vi "Settings_dialog.vi"(11 "Initial_cofig":path) -> (1 "canceled or no change?":bool, 3 "Settings":T1)   [LabVIEW 2012]
uses:
  controls/Video_analizer_settings.ctl
  <vilib>/Utility/config.llb/Read Key (Double).vi
  <vilib>/Utility/config.llb/Read Key (Boolean).vi
  <vilib>/Utility/config.llb/Read Key (U32).vi
  <vilib>/Utility/config.llb/NI_LVConfig.lvlib
panel:
  in  "Order":u32 caption="Порядок"
  in  "Cutof_freq":dbl caption="Частота среза, Гц"
  in  "FIR_enable":bool caption="Вкл. цифровой фильтр"
  in  "VoltageY_offset":dbl caption="Смещение по Y напряжения, В"
  in  "CurrentY_offset":dbl caption="Смещение по Y тока, А"
  in  "Video_shift_in":dbl caption="Смещение видео-напряжение, мкс" min=0.0
  in  "Current_shift_in":dbl caption="Смещение ток-напряжение, мкс" min=0.0
  in  "Cancel Button":bool
  in  "Save Button":bool
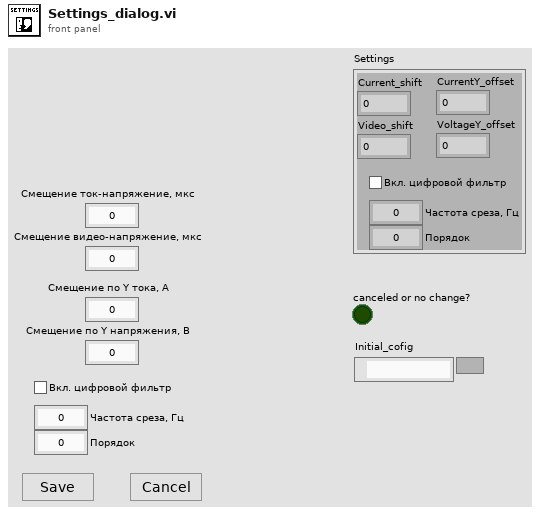
[diagram p1: front panel]
types:
  T1 = typedef "Video_analizer_settings.ctl" = cluster{"Current_shift":dbl, "Video_shift":dbl, "CurrentY_offset":dbl, "VoltageY_offset":dbl, "FIR_enable":bool, "Cutof_freq":dbl, "Order":u32}
  T2 = typedef "NI_LVConfig.lvlib/Config Data RefNum.ctl" = refnum<k1>
  T3 = enum8{"Enabled", "Disabled", "Disabled and Grayed Out"}
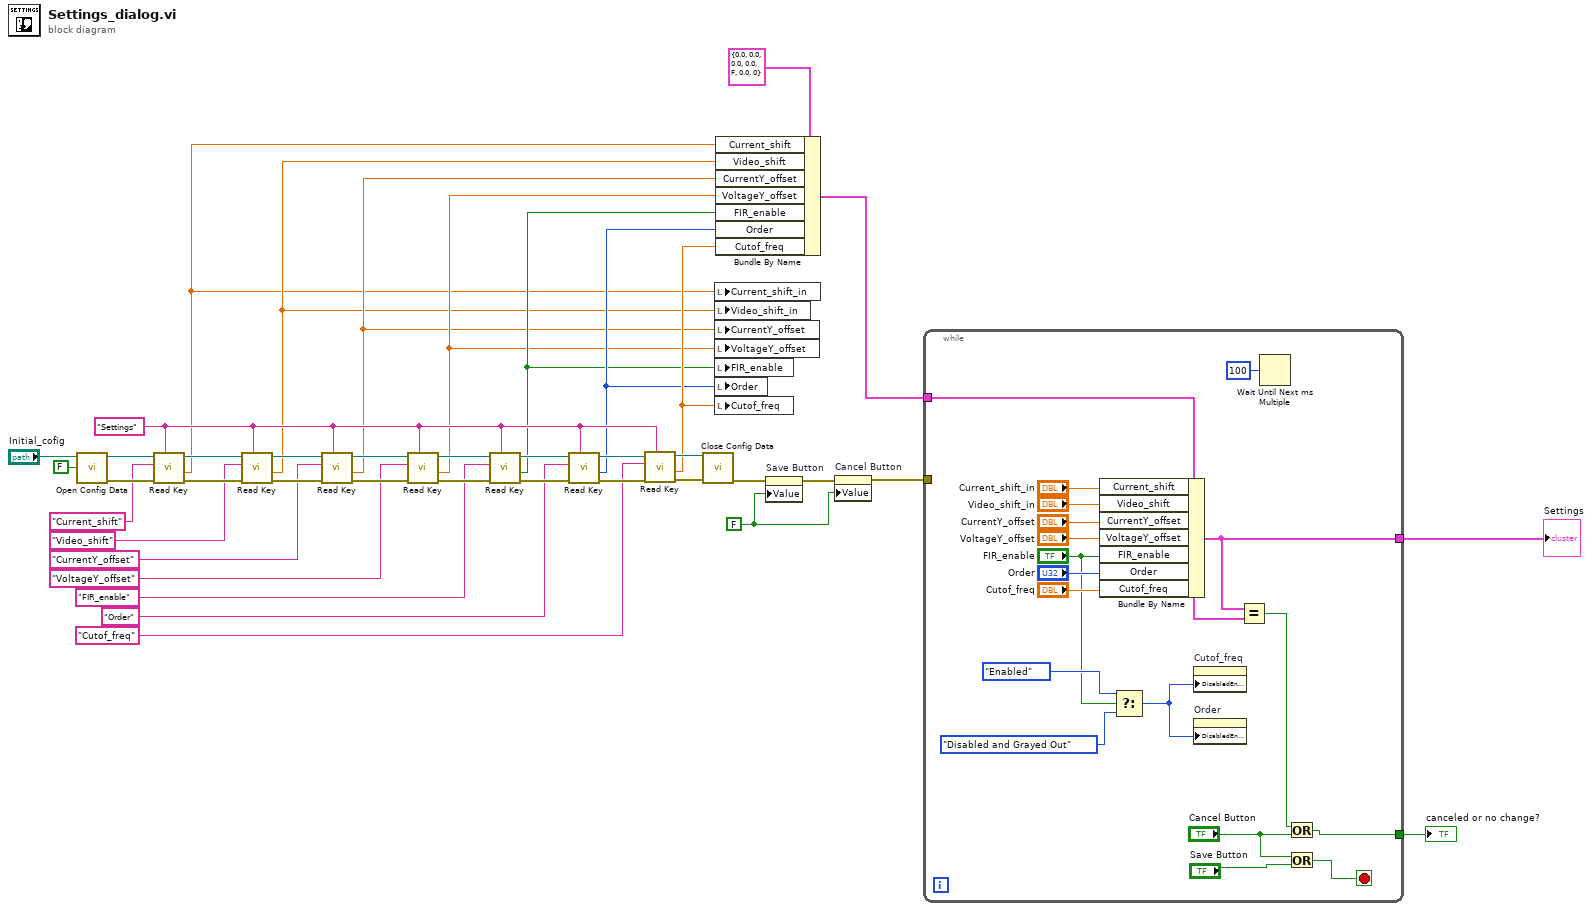
[diagram p0: block diagram]
diagram:
  w13 = "Settings" ("section")
  w39 = FALSE ("Save Button")
  n1 = call <vilib>:"Open Config Data.vi"("create file if necessary (T)"=FALSE, "configuration file path"="Initial_cofig") -> ("error out"=w32:errorcluster, "refnum"=w35:T2)  [unwired: 7 in, 1 out]
  n2 = call-poly <vilib>:"Read Key.vi"("section"=w13, "error in (no error)"=w32, "key"="Current_shift", "refnum"=w35) -> ("error out"=w33:errorcluster, "value"=w3:dbl, "refnum out"=w34:T2)  [unwired: 4 in, 1 out]
  n3 = call-poly <vilib>:"Read Key.vi"("section"=w13, "error in (no error)"=w33, "key"="Video_shift", "refnum"=w34) -> ("error out"=w26:errorcluster, "value"=w4:dbl, "refnum out"=w28:T2)  [unwired: 4 in, 1 out]
  n4 = call-poly <vilib>:"Read Key.vi"("section"=w13, "error in (no error)"=w26, "key"="CurrentY_offset", "refnum"=w28) -> ("error out"=w25:errorcluster, "value"=w5:dbl, "refnum out"=w27:T2)  [unwired: 4 in, 1 out]
  n5 = call-poly <vilib>:"Read Key.vi"("section"=w13, "error in (no error)"=w25, "key"="VoltageY_offset", "refnum"=w27) -> ("error out"=w21:errorcluster, "value"=w6:dbl, "refnum out"=w17:T2)  [unwired: 4 in, 1 out]
  n6 = call-poly <vilib>:"Read Key.vi"("section"=w13, "error in (no error)"=w21, "key"="FIR_enable", "refnum"=w17) -> ("error out"=w20:errorcluster, "value"=w7:bool, "refnum out"=w16:T2)  [unwired: 4 in, 1 out]
  n7 = call-poly <vilib>:"Read Key.vi"("section"=w13, "error in (no error)"=w20, "key"="Order", "refnum"=w16) -> ("error out"=w19:errorcluster, "value"=w8:u32, "refnum out"=w15:T2)  [unwired: 4 in, 1 out]
  n8 = call-poly <vilib>:"Read Key.vi"("section"=w13, "error in (no error)"=w19, "key"="Cutof_freq", "refnum"=w15) -> ("error out"=w18:errorcluster, "value"=w9:dbl, "refnum out"=w14:T2)  [unwired: 4 in, 1 out]
  n9 = call <vilib>:"Close Config Data.vi"("error in (no error)"=w18, "refnum"=w14) -> ("error out"=w29:errorcluster)  [unwired: 8 in, 1 out]
  n10 = local write "Current_shift_in"(w3) -> ()
  n11 = local write "Video_shift_in"(w4) -> ()
  n12 = local write "CurrentY_offset"(w5) -> ()
  n13 = local write "VoltageY_offset"(w6) -> ()
  n14 = local write "FIR_enable"(w7) -> ()
  n15 = local write "Order"(w8) -> ()
  n16 = local write "Cutof_freq"(w9) -> ()
  n17 = Bundle By Name(cluster=T1 {"Current_shift"=0.0, "Video_shift"=0.0, "CurrentY_offset"=0.0, "VoltageY_offset"=0.0, "FIR_enable"=FALSE, "Cutof_freq"=0.0, "Order"=0} ("Settings"), "Current_shift"=w3, "Video_shift"=w4, "CurrentY_offset"=w5, "VoltageY_offset"=w6, "FIR_enable"=w7, "Order"=w8, "Cutof_freq"=w9) -> (w2:T1)
  n18 = property on="Save Button" class="Bool (strict)"(error in=w29, "Value"=w39) -> (error out=w41:errorcluster)  [unwired: 1 in, 1 out]
  n19 = property on="Cancel Button" class="Bool (strict)"(error in=w41, "Value"=w39) -> (error out=w40:errorcluster)  [unwired: 1 in, 1 out]
  n20 = while {
    tunnel: w40 -> [_]
    tunnel: [w55] -> w38
    tunnel: w2 -> [w47]
    tunnel: [w48] -> w1
    stop <- w57 stop-if-true
    n21 = Bundle By Name(cluster=w47, "Current_shift"="Current_shift_in", "Video_shift"="Video_shift_in", "CurrentY_offset"="CurrentY_offset", "VoltageY_offset"="VoltageY_offset", "FIR_enable"="FIR_enable", "Order"="Order", "Cutof_freq"="Cutof_freq") -> (w48:T1)
    n22 = Select(t=T3."Enabled" ("Disabled"), s="FIR_enable", f=T3."Disabled and Grayed Out" ("Disabled")) -> (s? t:f=w42:T3)
    n23 = property on="Cutof_freq" class="DigNum (strict)"("DisabledEnum"=w42) -> ()  [unwired: 2 in, 2 out]
    n24 = property on="Order" class="DigNum (strict)"("DisabledEnum"=w42) -> ()  [unwired: 2 in, 2 out]
    n25 = Equal?(x=w48, y=w47) -> (x = y?=w46:bool)
    n26 = Wait Until Next ms Multiple(millisecond multiple=u32 100) -> ()  [unwired: 1 out]
    n27 = Or(x=w46, y="Cancel Button") -> (x .or. y?=w55:bool)
    n28 = Or(x="Cancel Button", y="Save Button") -> (x .or. y?=w57:bool)
  }
  "canceled or no change?" <- w38
  "Settings" <- w1
